vi "InterpretForLoop.vi"(5 "Loop in":refnum<class "Loop.lvclass">, 6 "error in":errorcluster, 9 "VI Interpreter in":refnum<class "VI Interpreter.lvclass">) -> (0 "error out":errorcluster, 3 "VI Interpreter out":refnum<class "VI Interpreter.lvclass">, 4 "Loop out":refnum<class "Loop.lvclass">)   [LabVIEW 2014, in "VI Interpreter.lvclass"]
uses:
  VI Interpreter.lvclass
  Loop/Loop.lvclass
  ForLoop/ForLoop.lvclass
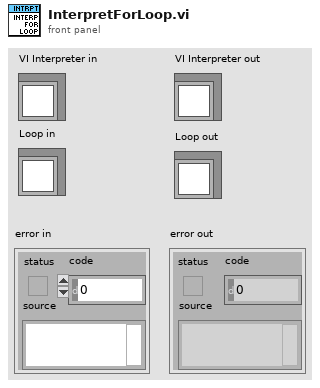
[diagram p1: front panel]
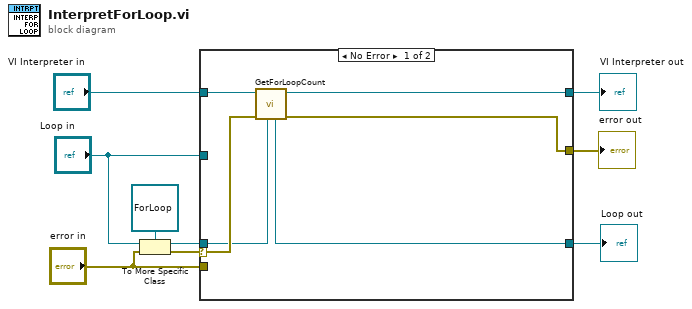
[diagram p0: block diagram]
diagram:
  n1 = To More Specific Class(target class=refnum<class "ForLoop.lvclass"> refnum ("Loop in"), reference="Loop in", error in="error in") -> (specific class reference=w4:refnum<class "ForLoop.lvclass">, error out=w3:errorcluster)
  n2 = case shown="No Error" w3 {
    selector: w3 -> [w14 _]
    tunnel: "VI Interpreter in" -> [w15 w17]
    tunnel: [w12 w16] -> w8
    tunnel: [w10 w17] -> w7
    tunnel: [w13 w18] -> w6
    tunnel: w4 -> [w11 _]
    tunnel: "error in" -> [_ w18]
    tunnel: "Loop in" -> [_ w16]
    frame No Error {
      n3 = call "GetForLoopCount.vi"("ForLoop in"=w11, "error in"=w14, "VI Interpreter in"=w15) -> ("error out"=w13:errorcluster, "VI Interpreter out"=w10:refnum<class "VI Interpreter.lvclass">, "ForLoop out"=w12:refnum<class "ForLoop.lvclass">)  [unwired: 4 in]
    }
    frame Error {
    }
  }
  "error out" <- w6
  "VI Interpreter out" <- w7
  "Loop out" <- w8
